vi "POST Batch Details.vi"(0 "GTron in":path, 11 "error in":errorcluster) -> (4 "IsEmpty":bool, 15 "error out":errorcluster)   [LabVIEW 2019, in "DataLogger.lvclass"]
doc: "POST Batch Details"
uses:
  DataLogger.lvclass
  <vilib>/drjdpowell/SQLite Library/SQL Connection/Execute SQL (Single Integer).vi
  <vilib>/httpClient/LabVIEWHTTPClient.lvlib
  <vilib>/drjdpowell/SQLite Library/SQL Statement/SQL Statement.lvclass
  <vilib>/drjdpowell/SQLite Library/SQL Connection/Execute SQL (No results).vi
  <vilib>/drjdpowell/SQLite Library/SQL Connection/Open (path).vi
  <vilib>/httpClient/POSTBuffer.vi
  <vilib>/drjdpowell/SQLite Library/SQL Connection/Connection.lvclass
panel:
  in  "Server info Cluster for Reel in":T1={"JSON Buffer"="authtoken=47244d7c61d7e6141acdddeabbf622d1&scope=creatorapi&zc_ownername=zentron3&XMLString=", "Server information start tag"="<ZohoCreator> <applicationlist> <application name='iiot-gtron'><formlist>  <form name='SimulatedReelDetails'>", "Record start/end"="add", "Key name"="field name", "Value name"="value", "Server information end tag"="\"</form></formlist></application></applicationlist></ZohoCreator>"}
  in  "Reel Keys in":string[](array[string])=["BatchId", "PartName", "StampingMcId", "InspectionMcId", "OperatorName", "BatchCount", "BatchPassCount", "BatchFailCount"]
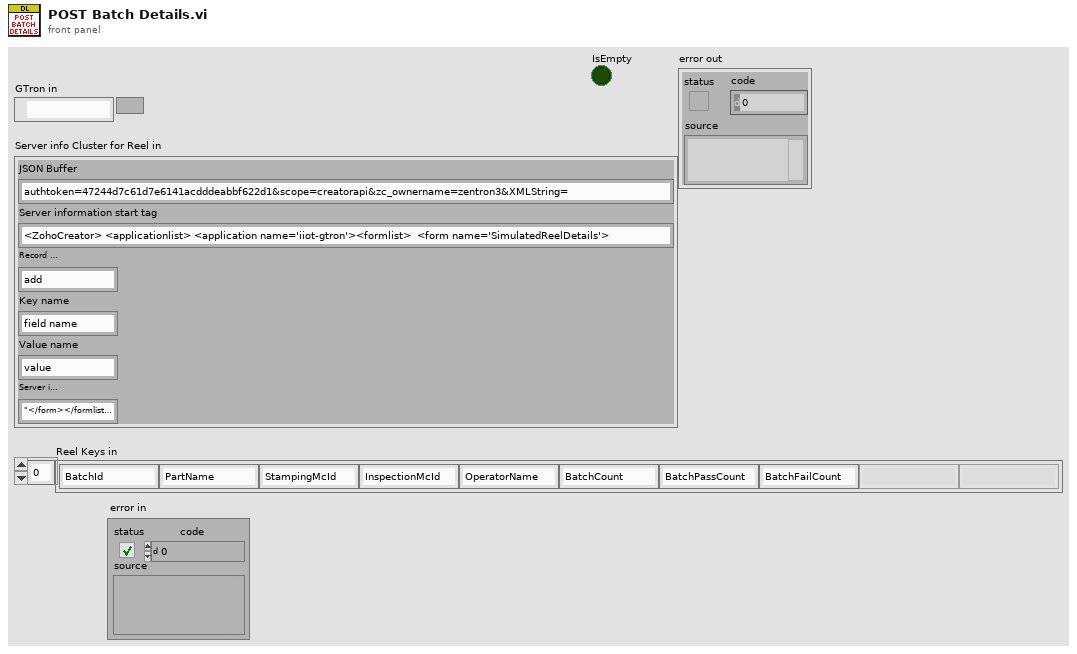
[diagram p1: front panel]
types:
  T1 = cluster{"JSON Buffer":string, "Server information start tag":string, "Record start/end":string, "Key name":string, "Value name":string, "Server information end tag":string}
  T2 = typedef "LabVIEWHTTPClient.lvlib/ClientHandle.ctl" = refnum<k1>
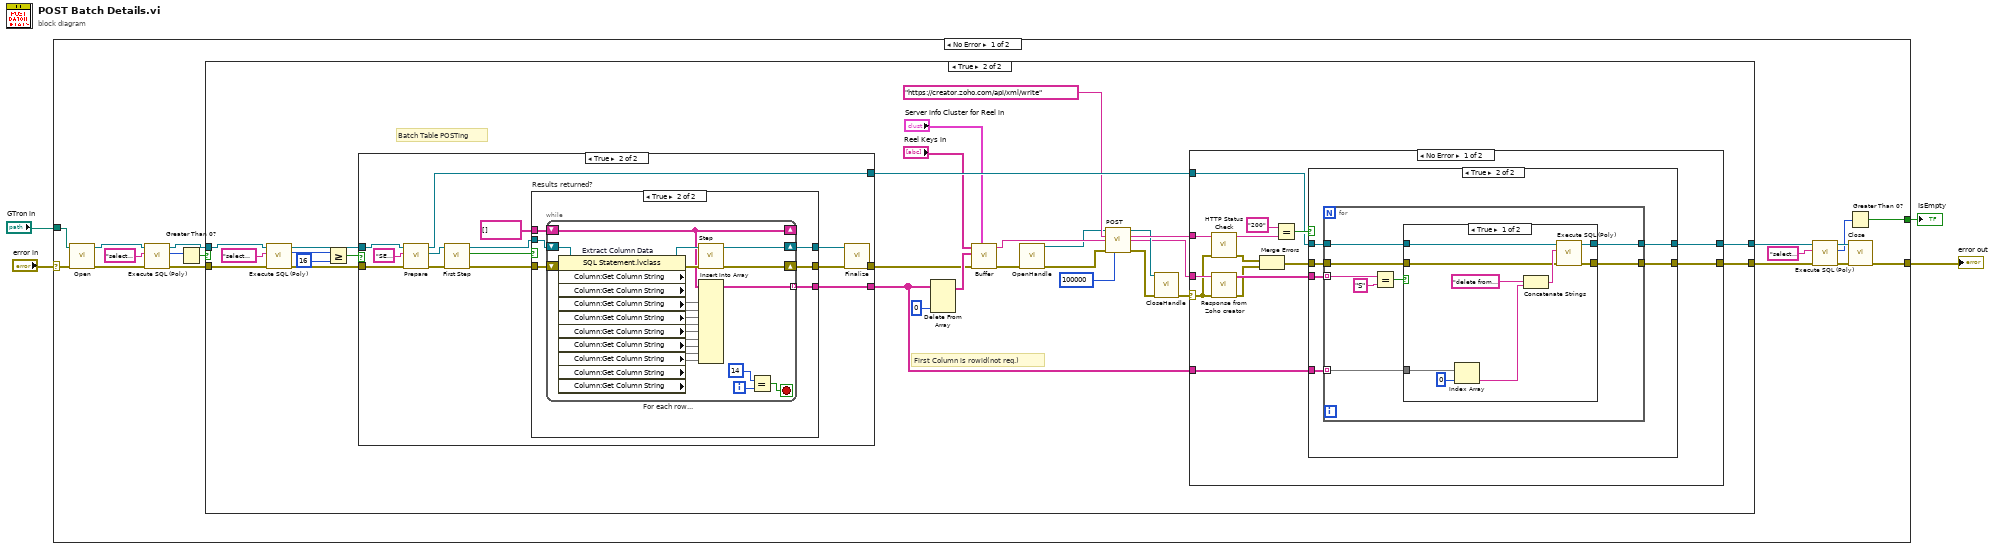
[diagram p0: block diagram]
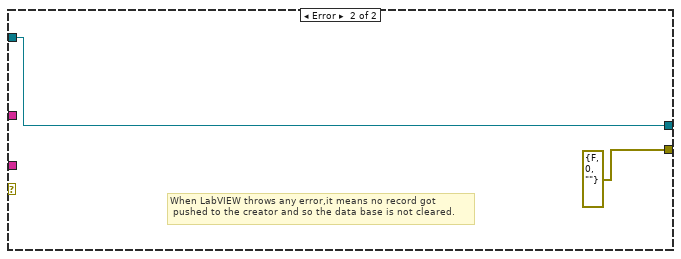
[diagram p5: hidden frame]
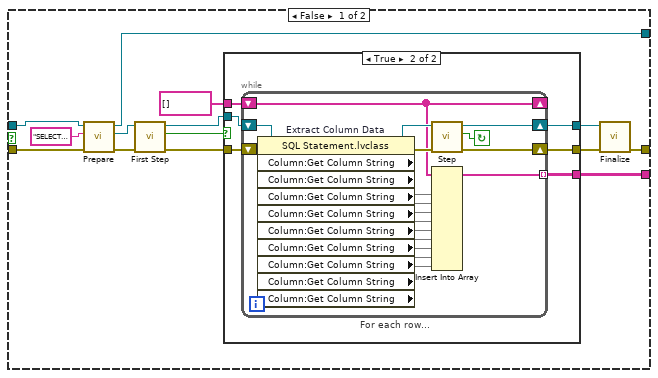
[diagram p6: hidden frame]
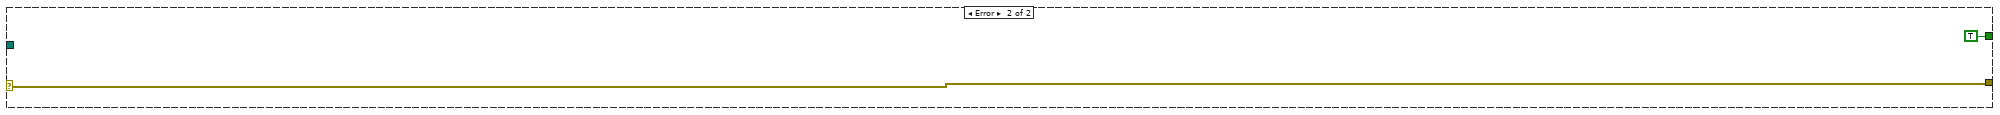
[diagram p9: hidden frame]
diagram:
  n1 = case shown="No Error" "error in" {
    selector: "error in" -> [w13 w178]
    tunnel: "GTron in" -> [w21 _]
    tunnel: [w8 w178] -> w3
    tunnel: [w6 TRUE] -> w1
    frame No Error {
      n2 = call-poly <vilib>:"Open.vi"("error in (no error)"=w13, "db file"=w21) -> ("error out"=w18:errorcluster, "SQLite Connection"=w19:refnum<class "Connection.lvclass">)  [unwired: 8 in]
      n3 = call-poly <vilib>:"Execute SQL (Poly).vi"("error in (no error)"=w18, "SQL"="select count(*) from BatchDetails ", "SQLite Connection in"=w19) -> ("error out"=w16:errorcluster, "Result"=w14:i64, "SQLite Connection"=w17:refnum<class "Connection.lvclass">)  [unwired: 6 in]
      n4 = Greater Than 0?(x=w14) -> (x > 0?=w15:bool)
      n5 = case shown="True" w15 {
        tunnel: [w22 w51] -> w7
        tunnel: [w23 w26] -> w9
        tunnel: w17 -> [w22 w25]
        tunnel: w16 -> [w23 w24]
        frame False {
        }
        frame True {
          # "Batch Table POSTing"
          # "First Column is rowid(not req.)"
          n6 = call-poly <vilib>:"Execute SQL (Poly).vi"("error in (no error)"=w24, "SQL"="select count(*) from BatchDetails ", "SQLite Connection in"=w25) -> ("error out"=w30:errorcluster, "Result"=w32:i64, "SQLite Connection"=w48:refnum<class "Connection.lvclass">)  [unwired: 6 in]
          n7 = Greater Or Equal?(x=w32, y=i64 16) -> (x >= y?=w34:bool)
          n8 = case shown="True" w34 {
            tunnel: [w100 w140] -> w50
            tunnel: w48 -> [w99 w139]
            tunnel: [w98 w138] -> w49
            tunnel: w30 -> [w96 w136]
            tunnel: [w95 w135] -> w29
            frame False {
              n9 = call <vilib>:"Prepare.vi"("error in (no error)"=w96, "SQL"="SELECT rowid,BatchID,PartName,StampingMcId,InspectionMcId,OperatorName,BatchCount,BatchPassCount,BatchFailCount FROM BatchDetails" ("SELECT  statement"), "SQLite Connection in"=w99) -> ("error out"=w107:errorcluster, "SQL Statement"=w103:refnum<class "SQL Statement.lvclass">, "SQLite Connection"=w98:refnum<class "Connection.lvclass">)  [unwired: 4 in, 2 out]
              n10 = call <vilib>:"First Step.vi"("error in (no error)"=w107, "SQL Statement in"=w103) -> ("error out"=w105:errorcluster, "Row returned"=w106:bool, "SQL Statement"=w104:refnum<class "SQL Statement.lvclass">)  [unwired: 7 in]
              n11 = case "Results returned?" shown="True" w106 {
                tunnel: [w110 w116] -> w102
                tunnel: [w109 w115] -> w101
                tunnel: w104 -> [w110 w114]
                tunnel: w105 -> [w109 w113]
                tunnel: string[] [] -> [_ w112]
                tunnel: [_ w111] -> w100
                frame False {
                }
                frame True {
                  n12 = while "For each row..." {
                    shift-right: [w133] -> w116
                    shift-left: w114 -> [w130]
                    shift-right: [w131] -> w115
                    shift-left: w113 -> [w129]
                    shift-right: [w128] -> _
                    shift-left: w112 -> [w128]
                    tunnel: [w120] -> w111 mode=indexing
                    stop <- w118 continue-if-true
                    n13 = property on="Extract Column Data" class="SQL Statement.lvclass"(reference=w130, error in=w129) -> (reference out=w134:refnum<class "SQL Statement.lvclass">, error out=w132:errorcluster, "Column:Get Column String"=w119, "Column:Get Column String"=w127, "Column:Get Column String"=w126, "Column:Get Column String"=w125, "Column:Get Column String"=w124, "Column:Get Column String"=w123, "Column:Get Column String"=w122, "Column:Get Column String"=w121, "Column:Get Column String"=w117)
                    n14 = call <vilib>:"Step.vi"("error in (no error)"=w132, "SQL Statement in"=w134) -> ("error out"=w131:errorcluster, "Row returned"=w118:bool, "SQL Statement"=w133:refnum<class "SQL Statement.lvclass">)  [unwired: 7 in]
                    n15 = Insert Into Array(array=w128, new element #1=w119, new element #2=w127, new element #3=w126, new element #4=w125, new element #5=w124, new element #6=w123, new element #7=w122, new element #8=w121, new element #9=w117) -> (w120:string[])  [unwired: 1 in]
                  }
                }
              }
              n16 = call <vilib>:"Finalize.vi"("error in (no error)"=w101, "SQL Statement in"=w102) -> ("error out"=w95:errorcluster)  [unwired: 9 in]
            }
            frame True {
              n17 = call <vilib>:"Prepare.vi"("error in (no error)"=w136, "SQL"="SELECT rowid,BatchID,PartName,StampingMcId,InspectionMcId,OperatorName,BatchCount,BatchPassCount,BatchFailCount FROM BatchDetails" ("SELECT  statement"), "SQLite Connection in"=w139) -> ("error out"=w147:errorcluster, "SQL Statement"=w143:refnum<class "SQL Statement.lvclass">, "SQLite Connection"=w138:refnum<class "Connection.lvclass">)  [unwired: 4 in, 2 out]
              n18 = call <vilib>:"First Step.vi"("error in (no error)"=w147, "SQL Statement in"=w143) -> ("error out"=w145:errorcluster, "Row returned"=w146:bool, "SQL Statement"=w144:refnum<class "SQL Statement.lvclass">)  [unwired: 7 in]
              n19 = case "Results returned?" shown="True" w146 {
                tunnel: [w150 w156] -> w142
                tunnel: [w149 w155] -> w141
                tunnel: w144 -> [w150 w154]
                tunnel: w145 -> [w149 w153]
                tunnel: string[] [] -> [_ w152]
                tunnel: [_ w151] -> w140
                frame False {
                }
                frame True {
                  n20 = while "For each row..." {
                    shift-right: [w175] -> w156
                    shift-left: w154 -> [w172]
                    shift-right: [w173] -> w155
                    shift-left: w153 -> [w171]
                    shift-right: [w170] -> _
                    shift-left: w152 -> [w170]
                    tunnel: [w162] -> w151 mode=indexing
                    i -> [w161]
                    stop <- w159 stop-if-true
                    n21 = property on="Extract Column Data" class="SQL Statement.lvclass"(reference=w172, error in=w171) -> (reference out=w176:refnum<class "SQL Statement.lvclass">, error out=w174:errorcluster, "Column:Get Column String"=w158, "Column:Get Column String"=w169, "Column:Get Column String"=w168, "Column:Get Column String"=w167, "Column:Get Column String"=w166, "Column:Get Column String"=w165, "Column:Get Column String"=w164, "Column:Get Column String"=w163, "Column:Get Column String"=w157)
                    n22 = call <vilib>:"Step.vi"("error in (no error)"=w174, "SQL Statement in"=w176) -> ("error out"=w173:errorcluster, "SQL Statement"=w175:refnum<class "SQL Statement.lvclass">)  [unwired: 7 in, 1 out]
                    n23 = Insert Into Array(array=w170, new element #1=w158, new element #2=w169, new element #3=w168, new element #4=w167, new element #5=w166, new element #6=w165, new element #7=w164, new element #8=w163, new element #9=w157) -> (w162:string[])  [unwired: 1 in]
                    n24 = Equal?(x=14, y=w161) -> (x = y?=w159:bool)
                  }
                }
              }
              n25 = call <vilib>:"Finalize.vi"("error in (no error)"=w141, "SQL Statement in"=w142) -> ("error out"=w135:errorcluster)  [unwired: 9 in]
            }
          }
          n26 = Delete From Array(array=w50, index (col)=0 ("disabled index (col)")) -> (array with subset deleted=w36:string[][])  [unwired: 2 in, 1 out]
          n27 = call "Buffer.vi"("Cluster"="Server info Cluster for Reel in", "error in"=w29, "Values"=w36, "Keys"="Reel Keys in") -> ("Error out"=w28:errorcluster, "Buffer"=w41:string)  [unwired: 6 in]
          n28 = call <vilib>:"OpenHandle.vi"("error in (no error)"=w28) -> ("client handle out"=w39:T2, "error out"=w44:errorcluster)  [unwired: 13 in]
          n29 = call-poly <vilib>:"POST.vi"("client handle"=w39, "url"="https://creator.zoho.com/api/xml/write", "buffer"=w41, "error in (no error)"=w44, "timeout (10000)"=100000) -> ("client handle out"=w40:T2, "headers"=w47:string, "body"=w27:string, "error out"=w45:errorcluster)  [unwired: 7 in]
          n30 = call <vilib>:"CloseHandle.vi"("client handle"=w40, "error in (no error)"=w45) -> ("error out"=w46:errorcluster)  [unwired: 13 in]
          n31 = case shown="No Error" w46 {
            selector: w46 -> [w56 _]
            tunnel: w47 -> [w65 _]
            tunnel: w27 -> [w58 _]
            tunnel: w49 -> [w61 w94]
            tunnel: w50 -> [w60 _]
            tunnel: [w59 w94] -> w51
            tunnel: [w52 errorcluster {"status"=FALSE, "code"=0, "source"=""} ("error out")] -> w26
            frame No Error {
              n32 = call "HTTP Status Check.vi"("error in (no error)"=w56, "String"=w65) -> ("error out"=w55:errorcluster, "HTTP Status Code"=w64:string)  [unwired: 7 in]
              n33 = call "Response from Zoho creator.vi"("error in"=w56, "body"=w58) -> ("error out"=w54:errorcluster, "decimated array"=w57:string[])  [unwired: 8 in]
              n34 = Merge Errors(w55, w54) -> (w53:errorcluster)
              n35 = Equal?(x="200" ("y"), y=w64) -> (x = y?=w62:bool)
              n36 = case shown="True" w62 {
                tunnel: w57 -> [_ w72]
                tunnel: w61 -> [w67 w73]
                tunnel: w60 -> [_ w71]
                tunnel: [w67 w70] -> w59
                tunnel: w53 -> [w66 w69]
                tunnel: [w66 w68] -> w52
                frame False {
                  # "When HTTP Status is anything except 200,it means no record\ngot pushed to the creator and so the database is not cleared"
                }
                frame True {
                  n37 = for {
                    tunnel: w73 -> [w81]
                    tunnel: w71 -> [w77] mode=indexing
                    tunnel: w72 -> [w80] mode=indexing
                    tunnel: [w76] -> w70
                    tunnel: w69 -> [w75]
                    tunnel: [w74] -> w68
                    n38 = Equal?(x=w80, y="S") -> (x = y?=w78:bool)
                    n39 = case shown="True" w78 {
                      tunnel: w81 -> [w90 w92]
                      tunnel: w77 -> [w89 _]
                      tunnel: [w84 w92] -> w76
                      tunnel: w75 -> [w83 w91]
                      tunnel: [w82 w91] -> w74
                      frame True {
                        n40 = Index Array(array=w89, index=0) -> (element=w87:string)
                        n41 = Concatenate Strings("delete from BatchDetails where rowid = " ("SQL"), w87) -> (w85:string)
                        n42 = call-poly <vilib>:"Execute SQL (Poly).vi"("error in (no error)"=w83, "SQL"=w85, "SQLite Connection in"=w90) -> ("error out"=w82:errorcluster, "SQLite Connection"=w84:refnum<class "Connection.lvclass">)  [unwired: 7 in]
                      }
                      frame False {
                      }
                    }
                  }
                }
              }
            }
            frame Error {
              # "When LabVIEW throws any error,it means no record got\n pushed to the creator and so the data base is not cleared."
            }
          }
        }
      }
      n43 = call-poly <vilib>:"Execute SQL (Poly).vi"("error in (no error)"=w9, "SQL"="select count(*) from BatchDetails ", "SQLite Connection in"=w7) -> ("error out"=w12:errorcluster, "Result"=w10:i64, "SQLite Connection"=w11:refnum<class "Connection.lvclass">)  [unwired: 6 in]
      n44 = Greater Than 0?(x=w10) -> (x > 0?=w6:bool)
      n45 = call-dynamic "Close.vi"("error in (no error)"=w12, "SQLite Connection in"=w11) -> ("error out"=w8:errorcluster)  [unwired: 9 in]
    }
    frame Error {
    }
  }
  "error out" <- w3
  "IsEmpty" <- w1
